vi "WPI_DigitalInputGetValue.vi"(8 "error in (no error)":errorcluster, 11 "DigitalInputDevRef":T1={"DevStatus"={"status"=FALSE, "code"=0, "source"=""}, "DIO Channel"=enum."Invalid"}) -> (0 "error out":errorcluster, 2 "Value":bool, 3 "DigitalInputDevRef":T1={"DevStatus"={"status"=FALSE, "code"=0, "source"=""}, "DIO Channel"=enum."Invalid"})   [LabVIEW 2017]
doc: "Returns the value of the digital input that you specify.\n\nThis software is licensed. Open the labview\\readme\\WPI Robotics Library Open Source License.txt file for more information."
uses:
  <vilib>/Rock Robotics/WPI/DigitalInput/WPI_DigitalInputDevRef.ctl
  <vilib>/Rock Robotics/SystemInterfaces/DIO/FPGA_DIOChannel.ctl
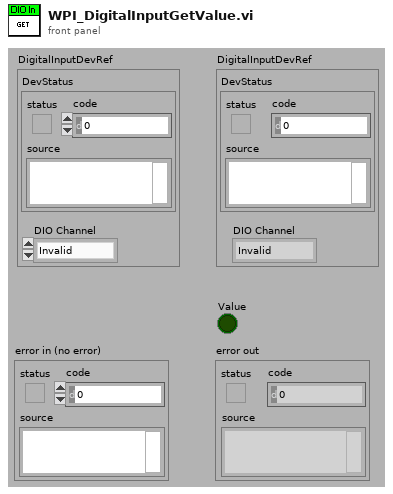
[diagram p1: front panel]
types:
  T1 = typedef "WPI_DigitalInputDevRef.ctl" = cluster{"DevStatus":errorcluster, "DIO Channel":T2}
  T2 = typedef "FPGA_DIOChannel.ctl" = enum8{"DIO 0", "DIO 1", "DIO 2", "DIO 3", "DIO 4", "DIO 5", "DIO 6", "DIO 7", "DIO 8", "DIO 9", "DIO MXP 0", "DIO MXP 1", "DIO MXP 2", "DIO MXP 3", "DIO MXP 4", "DIO MXP 5", "DIO MXP 6", "DIO MXP 7", "DIO MXP 8", "DIO MXP 9", "DIO MXP 10", "DIO MXP 11", "DIO MXP 12", "DIO MXP 13", "DIO MXP 14", "DIO MXP 15", "SPI Port CS1", "SPI Port CS2", "SPI Port CS3", "SPI Port MISO", "SPI Port MOSI", "Invalid"}
  T3 = typedef "WPI_DigitalModuleDeviceRef.ctl" = cluster{"DevStatus":errorcluster}
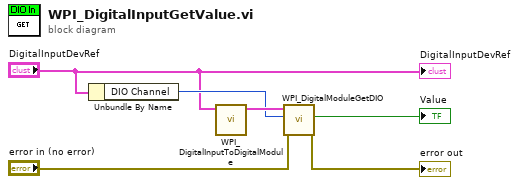
[diagram p0: block diagram]
diagram:
  n1 = Unbundle By Name("DigitalInputDevRef") -> ("DIO Channel"=w4:T2)
  n2 = call <vilib>:"WPI_DigitalInputToDigitalModule.vi"("DigitalInputDevRef"="DigitalInputDevRef") -> ("DigitalModuleDevRef"=w5:T3)  [unwired: 10 out]
  n3 = call <vilib>:"WPI_DigitalModuleGetDIO.vi"("error in (no error)"="error in (no error)", "DIOChannel"=w4, "DigitalModuleDevRef"=w5) -> ("error out"=→"error out":errorcluster, "Value"=→"Value":bool)  [unwired: 7 out]
  "DigitalInputDevRef" <- "DigitalInputDevRef"
